vi "Plot Robot.vi"(6 "Length":dbl, 9 "Angle":dbl, 10 "Location":cluster{"X":dbl, "Y":dbl}, 11 "Width":dbl) -> (3 "Cluster":cluster{"X Out":dbl[], "Y Out":dbl[]})   [LabVIEW 2019]
uses:
  <vilib>/Analysis/coordinate.llb/2D Cartesian Coordinate Rotation (Array).vi
  <vilib>/Analysis/coordinate.llb/2D Cartesian Coordinate Shift (Array).vi
  <vilib>/Analysis/NI_AALPro.lvlib
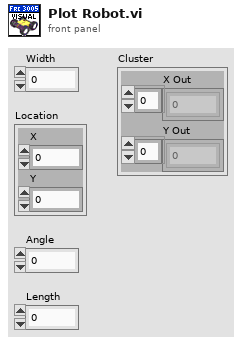
[diagram p1: front panel]
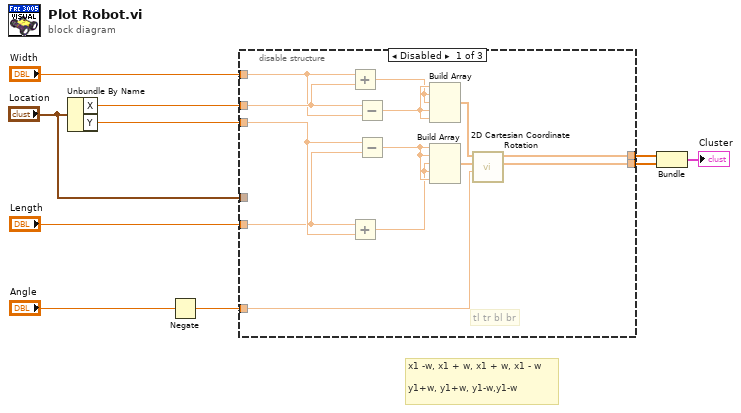
[diagram p0: block diagram]
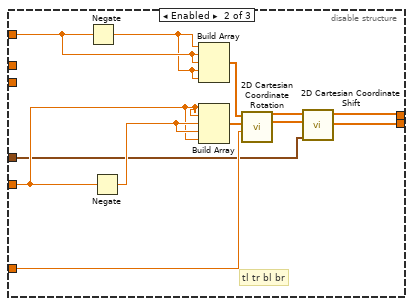
[diagram p2: hidden frame]
diagram:
  # "x1 -w, x1 + w, x1 + w, x1 - w\n\ny1+w, y1+w, y1-w,y1-w"
  n1 = Unbundle By Name("Location") -> ("X"=w3:dbl, "Y"=w5:dbl)
  n2 = Negate(x="Angle") -> (-x=w10:dbl)
  n3 = disable-structure shown="Disabled" {
    disable-tunnel: w10 -> [w23 w35 _]
    disable-tunnel: [w22 w25 _] -> w8
    disable-tunnel: [w21 w24 _] -> w7
    disable-tunnel: w5 -> [w14 _ _]
    disable-tunnel: "Length" -> [w13 w31 _]
    disable-tunnel: w3 -> [w12 _ _]
    disable-tunnel: "Width" -> [w11 w34 _]
    disable-tunnel: "Location" -> [_ w26 _]
    frame Disabled {
      # "tl tr bl br"
      n4 = Add(x=w11, y=w12) -> (x+y=w15:dbl)
      n5 = Add(x=w13, y=w14) -> (x+y=w16:dbl)
      n6 = Subtract(x=w12, y=w11) -> (x-y=w18:dbl)
      n7 = Subtract(x=w14, y=w13) -> (x-y=w17:dbl)
      n8 = Build Array(w18, w15, w15, w18, w18) -> (w19:dbl[])
      n9 = Build Array(w17, w17, w16, w16, w17) -> (w20:dbl[])
      n10 = call-poly <vilib>:"2D Cartesian Coordinate Rotation.vi"("theta"=w23, "Y"=w20, "X"=w19) -> ("Y Out"=w21:dbl[], "X Out"=w22:dbl[])  [unwired: 6 in, 1 out]
    }
    frame Enabled {
      # "tl tr bl br"
      n11 = Negate(x=w34) -> (-x=w33:dbl)
      n12 = Negate(x=w31) -> (-x=w32:dbl)
      n13 = Build Array(w33, w34, w34, w33, w33) -> (w30:dbl[])
      n14 = Build Array(w31, w31, w32, w32, w31) -> (w29:dbl[])
      n15 = call-poly <vilib>:"2D Cartesian Coordinate Rotation.vi"("theta"=w35, "Y"=w29, "X"=w30) -> ("Y Out"=w27:dbl[], "X Out"=w28:dbl[])  [unwired: 6 in, 1 out]
      n16 = call-poly <vilib>:"2D Cartesian Coordinate Shift.vi"("shift"=w26, "Y"=w27, "X"=w28) -> ("Y Out"=w24:dbl[], "X Out"=w25:dbl[])  [unwired: 6 in, 1 out]
    }
    frame Disabled {
    }
  }
  n17 = Bundle("X Out"=w8, "Y Out"=w7) -> (→"Cluster":cluster{"X Out":dbl[], "Y Out":dbl[]})  [unwired: 1 in]
